vi "VI Tree.vi"   [LabVIEW 2018, in "Keithley 2000.lvlib"]
doc: "This is the instrument driver for the Keithley 2000 Series instruments. The VI Tree displays all the user-callable VIs of the instrument driver in an organized table."
uses:
  <instrlib>/Keithley 2000/Keithley 2000.lvlib
  <instrlib>/Keithley 2000/Public/Configure/Configure Route Single.vi
panel:
  # "© 2003, National Instruments.  All Rights Reserved."
  # "SEE DIAGRAM\nFOR VI TREE."
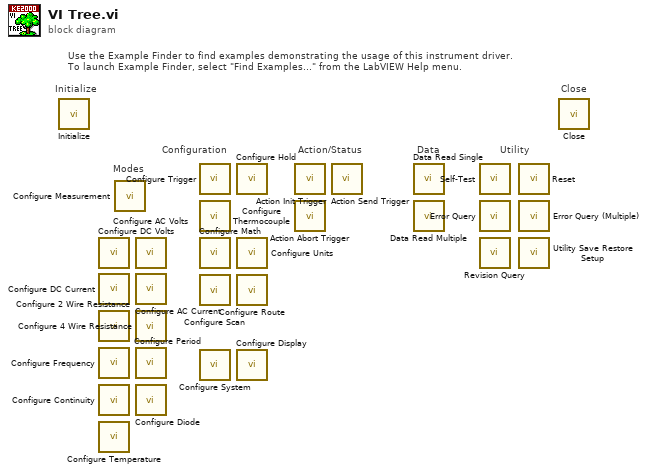
[diagram p0: block diagram]
diagram:
  # "Modes"
  # "Use the Example Finder to find examples demonstrating the usage of this instrument driver.\nTo launch Example Finder, select \"Find Examples...\" from the LabVIEW Help menu."
  # "Configuration"
  # "Utility"
  # "Data"
  # "Action/Status"
  # "Close"
  # "Initialize"
  n1 = call <instrlib>:"Initialize.vi"() -> ()  [unwired: 18 in, 2 out]
  n2 = call <instrlib>:"Configure DC Volts.vi"() -> ()  [unwired: 18 in, 2 out]
  n3 = call <instrlib>:"Configure DC Current.vi"() -> ()  [unwired: 18 in, 2 out]
  n4 = call <instrlib>:"Configure 2 Wire Resistance.vi"() -> ()  [unwired: 18 in, 2 out]
  n5 = call <instrlib>:"Configure Frequency.vi"() -> ()  [unwired: 18 in, 2 out]
  n6 = call <instrlib>:"Configure Continuity.vi"() -> ()  [unwired: 18 in, 2 out]
  n7 = call <instrlib>:"Configure Temperature.vi"() -> ()  [unwired: 18 in, 2 out]
  n8 = call-poly <instrlib>:"Configure Measurement.vi"() -> ()  [unwired: 18 in, 2 out]
  n9 = call <instrlib>:"Configure AC Volts.vi"() -> ()  [unwired: 18 in, 2 out]
  n10 = call <instrlib>:"Configure AC Current.vi"() -> ()  [unwired: 18 in, 2 out]
  n11 = call <instrlib>:"Configure 4 Wire Resistance.vi"() -> ()  [unwired: 18 in, 2 out]
  n12 = call <instrlib>:"Configure Period.vi"() -> ()  [unwired: 18 in, 2 out]
  n13 = call <instrlib>:"Configure Diode.vi"() -> ()  [unwired: 18 in, 2 out]
  n14 = call <instrlib>:"Configure Trigger.vi"() -> ()  [unwired: 18 in, 2 out]
  n15 = call <instrlib>:"Configure Thermocouple.vi"() -> ()  [unwired: 18 in, 2 out]
  n16 = call <instrlib>:"Configure Math.vi"() -> ()  [unwired: 18 in, 2 out]
  n17 = call <instrlib>:"Configure Scan.vi"() -> ()  [unwired: 18 in, 2 out]
  n18 = call <instrlib>:"Configure System.vi"() -> ()  [unwired: 18 in, 2 out]
  n19 = call <instrlib>:"Configure Hold.vi"() -> ()  [unwired: 18 in, 2 out]
  n20 = call <instrlib>:"Configure Units.vi"() -> ()  [unwired: 18 in, 2 out]
  n21 = call-poly <instrlib>:"Configure Route.vi"() -> ()  [unwired: 18 in, 2 out]
  n22 = call <instrlib>:"Configure Display.vi"() -> ()  [unwired: 18 in, 2 out]
  n23 = call <instrlib>:"Action Init Trigger.vi"() -> ()  [unwired: 18 in, 2 out]
  n24 = call <instrlib>:"Action Abort Trigger.vi"() -> ()  [unwired: 18 in, 2 out]
  n25 = call <instrlib>:"Action Send Trigger.vi"() -> ()  [unwired: 18 in, 2 out]
  n26 = call <instrlib>:"Data Read Single.vi"() -> ()  [unwired: 15 in, 5 out]
  n27 = call <instrlib>:"Data Read Multiple.vi"() -> ()  [unwired: 15 in, 5 out]
  n28 = call <instrlib>:"Self-Test.vi"() -> ()  [unwired: 16 in, 4 out]
  n29 = call <instrlib>:"Error Query.vi"() -> ()  [unwired: 16 in, 4 out]
  n30 = call <instrlib>:"Revision Query.vi"() -> ()  [unwired: 16 in, 4 out]
  n31 = call <instrlib>:"Reset.vi"() -> ()  [unwired: 18 in, 2 out]
  n32 = call <instrlib>:"Error Query (Multiple).vi"() -> ()  [unwired: 16 in, 4 out]
  n33 = call <instrlib>:"Utility Save Restore Setup.vi"() -> ()  [unwired: 18 in, 2 out]
  n34 = call <instrlib>:"Close.vi"() -> ()  [unwired: 19 in, 1 out]
